vi "DefenderNicolas.vi"(0 "R":dbl[](array[numeric]), 1 "Field":dbl[](array[numeric]), 2 "Ball":dbl[](array[numeric]), 3 "Numeric":dbl) -> (8 "target":dbl[](array[numeric]))   [LabVIEW 2016]
panel:
  in  "dis entre robos":i32=200
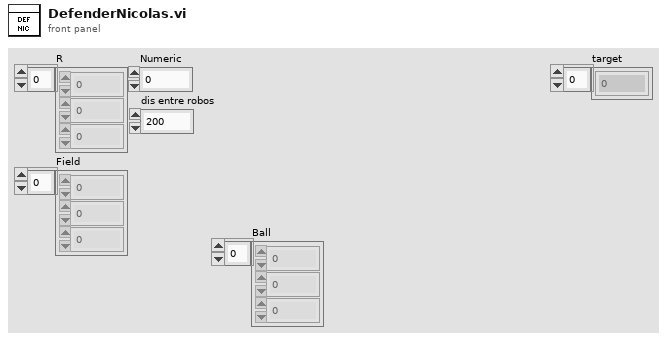
[diagram p1: front panel]
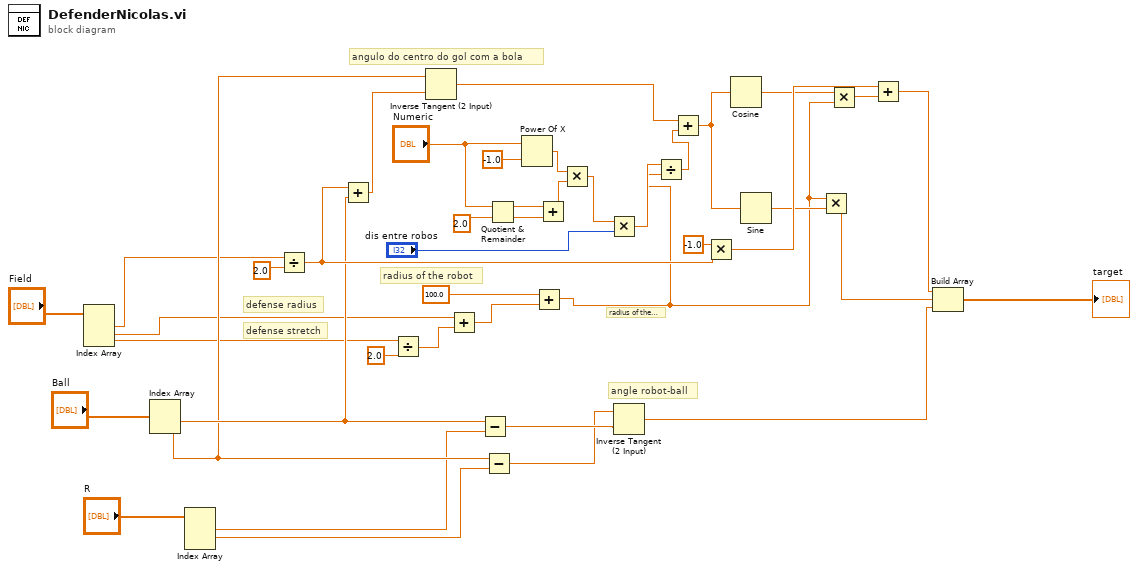
[diagram p0: block diagram]
diagram:
  # "angulo do centro do gol com a bola"
  # "defense stretch"
  # "defense radius"
  # "radius of the robot"
  # "angle robot-ball"
  # "radius of the circle"
  n1 = Index Array(array="Field") -> (element #1=w15:dbl, element #2=w21:dbl, element #3=w13:dbl)  [unwired: 3 in]
  n2 = Index Array(array="Ball") -> (element #1=w23:dbl, element #2=w22:dbl)  [unwired: 2 in]
  n3 = Index Array(array="R") -> (element #1=w16:dbl, element #2=w24:dbl)  [unwired: 3 in, 1 out]
  n4 = Divide(x=w15, y=2.0) -> (x/y=w31:dbl)
  n5 = Add(x=w31, y=w23) -> (x+y=w36:dbl)
  n6 = Divide(x=w13, y=2.0) -> (x/y=w40:dbl)
  n7 = Inverse Tangent (2 Input)(1:w36, 2:w22) -> (0:w4:dbl)
  n8 = Add(x=w21, y=w40) -> (x+y=w41:dbl)
  n9 = Subtract(x=w23, y=w16) -> (x-y=w26:dbl)
  n10 = Subtract(x=w22, y=w24) -> (x-y=w25:dbl)
  n11 = Quotient & Remainder(x="Numeric", y=2.0) -> (x-y*floor(x/y)=w30:dbl, floor(x/y)=w29:dbl)
  n12 = Power Of X(1:-1.0 ("y"), 2:"Numeric") -> (0:w38:dbl)
  n13 = Add(x=100.0, y=w41) -> (x+y=w2:dbl)
  n14 = Add(x=w30, y=w29) -> (x+y=w28:dbl)
  n15 = Multiply(x=w38, y=w28) -> (x*y=w39:dbl)
  n16 = Multiply(x=w39, y="dis entre robos") -> (x*y=w3:dbl)
  n17 = Inverse Tangent (2 Input)(1:w26, 2:w25) -> (0:w27:dbl)
  n18 = Divide(x=w3, y=w2) -> (x/y=w1:dbl)
  n19 = Add(x=w4, y=w1) -> (x+y=w37:dbl)
  n20 = Multiply(x=-1.0 ("y"), y=w31) -> (x*y=w42:dbl)
  n21 = Cosine(x=w37) -> (cos(x)=w34:dbl)
  n22 = Sine(x=w37) -> (sin(x)=w8:dbl)
  n23 = Multiply(x=w2, y=w8) -> (x*y=w33:dbl)
  n24 = Multiply(x=w34, y=w2) -> (x*y=w9:dbl)
  n25 = Add(x=w42, y=w9) -> (x+y=w35:dbl)
  n26 = Build Array(w35, w33, w27) -> (→"target":dbl[])
